vi "Open.vi"(8 "error in (no error)":errorcluster, 11 "TCatAdsNet in":refnum<class "AdsNET.lvclass">) -> (0 "error out":errorcluster, 3 "TCatAdsNet out":refnum<class "AdsNET.lvclass">)   [LabVIEW 2016, in "TCatAdsNet.lvlib" / "AdsNET.lvclass"]
doc: "Establishes a connection to a ADS device."
uses:
  AdsNET.lvclass
  C:/Users/Maurizio/Projects/twincat-lv-ads-library/TCatAdsNet Library/TwinCAT.Ads.dll
  TwinCAT.Ads.dll
  AdsNET.lvclass/AdsNET.ctl
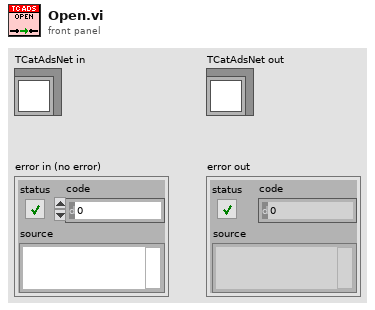
[diagram p1: front panel]
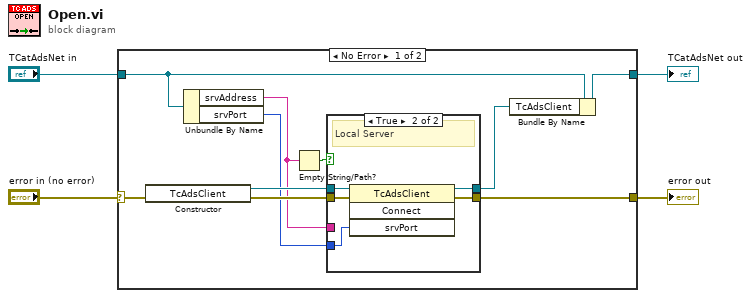
[diagram p0: block diagram]
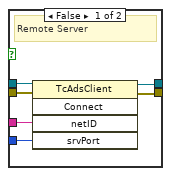
[diagram p2: hidden frame]
diagram:
  n1 = case shown="No Error" "error in (no error)" {
    selector: "error in (no error)" -> [w5 w26]
    tunnel: "TCatAdsNet in" -> [w12 w27]
    tunnel: [w10 w27] -> w3
    tunnel: [w8 w26] -> w2
    frame No Error {
      n2 = constructor class="TcAdsClient"(error in=w5) -> (reference out=w14:refnum<k24>, error out=w13:errorcluster)  [unwired: 2 in, 1 out]
      n3 = Unbundle By Name(w12) -> ("srvAddress"=w6:string, "srvPort"=w11:i32)
      n4 = Empty String/Path?(string/path=w6) -> (empty?=w7:bool)
      n5 = case shown="True" w7 {
        tunnel: w14 -> [w20 w25]
        tunnel: w13 -> [w19 w24]
        tunnel: w11 -> [w16 w23]
        tunnel: [w18 w22] -> w9
        tunnel: [w17 w21] -> w8
        tunnel: w6 -> [w15 _]
        frame False {
          # "Remote Server"
          n6 = invoke class="TcAdsClient" method="Connect"(reference=w20, error in=w19, "netID"=w15, "srvPort"=w16) -> (reference out=w18:refnum<k24>, error out=w17:errorcluster)  [unwired: 1 in, 3 out]
        }
        frame True {
          # "Local Server"
          n7 = invoke class="TcAdsClient" method="Connect"(reference=w25, error in=w24, "srvPort"=w23) -> (reference out=w22:refnum<k24>, error out=w21:errorcluster)  [unwired: 1 in, 2 out]
        }
      }
      n8 = Bundle By Name(cluster=w12, "TcAdsClient"=w9) -> (w10:refnum<class "AdsNET.lvclass">)
    }
    frame Error {
    }
  }
  "TCatAdsNet out" <- w3
  "error out" <- w2
